vi "Set Time Graph X Axis.vi"(8 "error in (no error)":errorcluster, 9 "End":timestamp, 10 "Start":timestamp, 11 "reference in":refnum<vi>) -> (0 "error out":errorcluster, 3 "reference out":refnum<vi>)   [LabVIEW 2016, in "Database Viewer.lvclass"]
uses:
  Database Viewer.lvclass
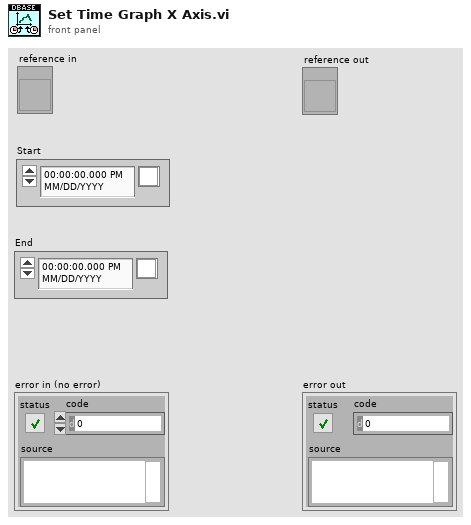
[diagram p1: front panel]
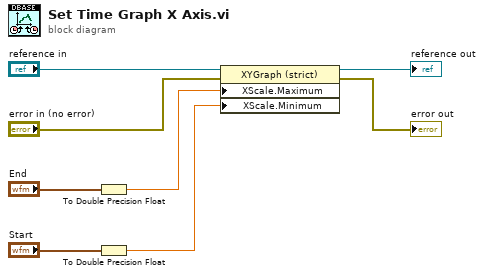
[diagram p0: block diagram]
diagram:
  n1 = To Double Precision Float(number="End") -> (double precision float=w6:dbl)
  n2 = To Double Precision Float(number="Start") -> (double precision float=w4:dbl)
  n3 = property on="Property Node" class="XYGraph (strict)"(reference="reference in", error in="error in (no error)", "XScale.Maximum"=w6, "XScale.Minimum"=w4) -> (reference out=→"reference out":refnum<vi>, error out=→"error out":errorcluster)
